vi "AI端口.vi"() -> ()   [LabVIEW 2013]
panel:
  out "AI端口":tag[](array[tag])=["Dev1/ai0", "Dev1/ai0", "Dev1/ai1", "Dev1/ai2", "Dev1/ai3"]
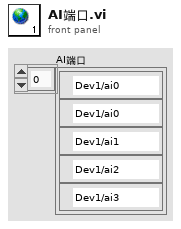
[diagram p1: front panel]
diagram:
